vi "SaveImageToFile.vi"(6 "strFilePath":u8[](array[numeric]), 8 "error in (no error)":errorcluster caption="错误输入（无错误）", 9 "pstSaveFileParam In":T1, 10 "handle":u64 format="%x", 11 "pData":u8[](array[numeric])) -> (0 "error out":errorcluster caption="错误输出", 1 "pstSaveFileParam Out":T1, 2 "handle out":u64 format="%x", 3 "function return":i32 format="%x")   [LabVIEW 2015, in "MvCameraControl.lvlib"]
doc: "MV_LV_API int __stdcall SaveImage(MV_SAVE_IMAGE_PARAM* pSaveParam);"
uses:
  MvCameraControl.lvlib
  MvCameraPatch.dll
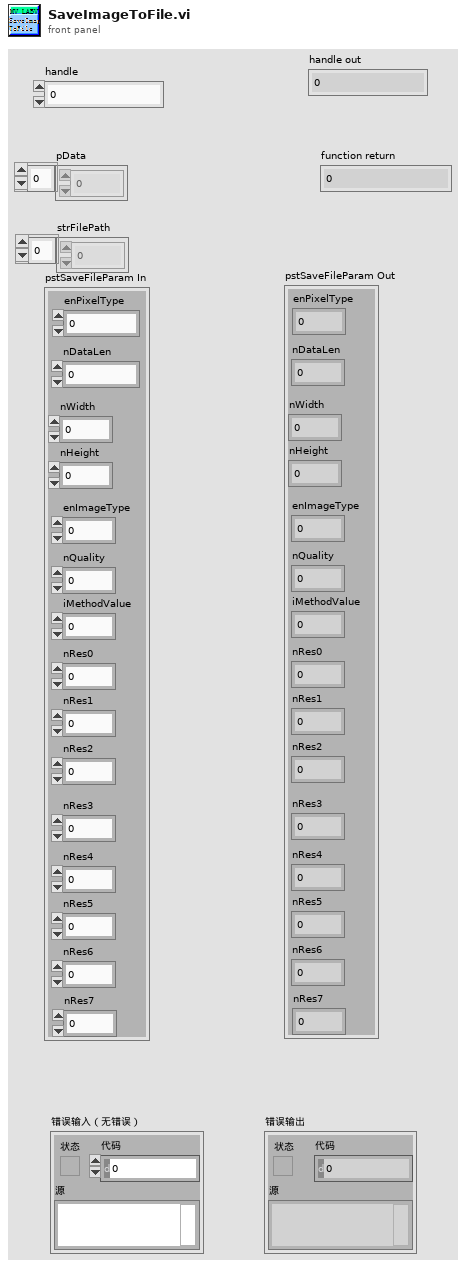
[diagram p1: front panel]
types:
  T1 = cluster{"enPixelType":i32, "nDataLen":u32, "nWidth":u16, "nHeight":u16, "enImageType":u32, "nQuality":u32, "iMethodValue":u32, "nRes0":u32, "nRes1":u32, "nRes2":u32, "nRes3":u32, "nRes6":u32, "nRes5":u32, "nRes4":u32, "nRes7":u32}
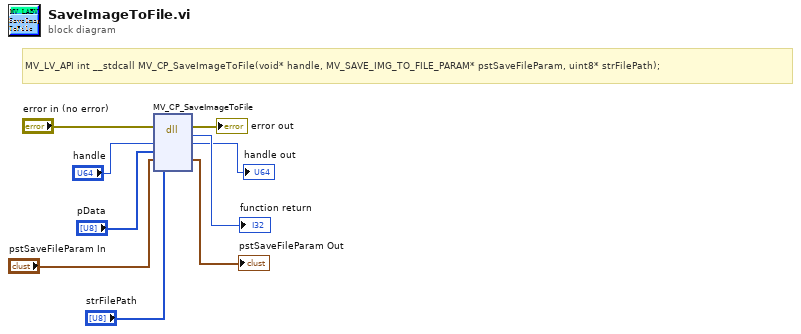
[diagram p0: block diagram]
diagram:
  # "MV_LV_API int __stdcall MV_CP_SaveImageToFile(void* handle, MV_SAVE_IMG_TO_FILE_PARAM* pstSaveFileParam, uint8* strFilePath);"
  n1 = dll-call lib="MvCameraPatch.dll" fn="MV_CP_SaveImageToFile"(error in="error in (no error)", "handle"="handle", "pData"="pData", "pstSaveFileParam"="pstSaveFileParam In", "strFilePath"="strFilePath") -> (error out=→"error out":errorcluster, "返回类型"=→"function return":i32, "handle"=→"handle out":u64, "pstSaveFileParam"=→"pstSaveFileParam Out":T1)  [unwired: 4 in, 1 out]
